vi "Swing-up Control.vi"() -> ()   [LabVIEW 2019]
uses:
  <vilib>/Simulation/Scripting/Companion Diagram/SimConfigNode/SimParams.ctl
  <vilib>/Simulation/Scripting/Companion Diagram/SimConfigNode/_simSolvers.ctl
  <vilib>/Simulation/Implementation/Shared/SIMSCR Execution Mode.ctl
  <vilib>/Platform/TimedLoop/XDataNode/timing_clust.ctl
  <vilib>/Platform/TimedLoop/XDataNode/nitl_modes.ctl
  <vilib>/Platform/TimedLoop/XDataNode/wakeup.ctl
  <vilib>/Simulation/Param Hierarchy/Typedefs/SIMPH Param Control Actions.ctl
  <vilib>/Simulation/Implementation/Shared/NILVSim_ParamChanged.vi
  <vilib>/Simulation/Implementation/Shared/NILVSim_FinishedLate.vi
  <vilib>/Simulation/Implementation/Shared/NILVSIM_BeginStep.vi
  <vilib>/Simulation/Utility/Implementation/SIM Halt.vi
  <vilib>/Simulation/DataSources/Implementation/NILVSim Signal Generator.llb/SIM Signal Generator (scalar).vi
  <vilib>/Simulation/SignalDisplay/Implementation/NILVSim Time Waveform.llb/SIM Time Waveform (vector).vi
  <vilib>/Simulation/SignalDisplay/Implementation/NILVSim Time Waveform.llb/SIM Time Waveform (scalar).vi
  <vilib>/Simulation/ContinuousLinear/Implementation/NILVSim Transfer Function Direct.llb/SIM Transfer Function Direct (SISO).vi
  <vilib>/Simulation/SignalArithmetic/Implementation/NILVSim Gain.llb/SIM Gain (dot product).vi
  <vilib>/Simulation/Nonlinear/Implementation/NILVSim Saturation.llb/SIM Saturation (scalar).vi
  <vilib>/Simulation/Implementation/Shared/NILVSim_Manager.vi
  <vilib>/Utility/error.llb/Clear Errors.vi
  <vilib>/Simulation/Implementation/Shared/NILVSim_FinalizeModel.vi
  <vilib>/Simulation/Implementation/Shared/SIM Unbundle Sim Info.vi
  <vilib>/Simulation/Implementation/Shared/SIMSH Read Queue.vi
  <vilib>/Simulation/Implementation/Shared/NILVSim_Initialize.vi
  SubVIs/Encoders.vi
  <vilib>/Simulation/Utility/Implementation/NILVSim Get Time and IsAcceptedStep.vi
  SubVIs/Motor.vi
  <vilib>/Simulation/Implementation/Shared/NILVSim_GetModelError.vi
  <vilib>/Simulation/Implementation/Shared/SIM Bundle Sim Info.vi
  <vilib>/Simulation/Scripting/Companion Diagram/SimConfigNode/SimDog.xnode
  SubVIs/Swing Up Energy Control.vi
  <vilib>/Platform/TimedLoop/XDataNode/XDataNode.xnode
  <vilib>/Simulation/Implementation/XNodeFramework/SimXNode/SimX.xnode
  <vilib>/Platform/TimedLoop/XDataNode/XDNodeRunTimeDep.lvlib
  <vilib>/Simulation/Implementation/Shared/NI_SIM_Implementation.lvlib
panel:
  in  "y":string="0"
  out "源端口":u16=65289
  out "源地址":u32=2887125761
  out "接收数据":string="0"
  out "错误输出 2":errorcluster caption="读取错误输出"
  out "错误输出":errorcluster caption="监听错误输出"
  in  "监听地址":string="192.168.8.144"
  in  "监听端口":u16=4096
  in  "Halt?":bool
  in  "Feedback Gain":dbl[](array[numeric])=[-3.39, 41.48, -1.38, 2.94]
  in  "Energy Control":T1={"Er (mJ)"=30.0, "mu (m/s^2/J)"=35.0, "u_max (m/s^2)"=6.0} {"u_max (m/s^2)" min=0.0 max=10.0 step=0.5; "mu (m/s^2/J)" min=0.0 max=150.0 step=5.0; "Er (mJ)" min=0.0 max=50.0 step=5.0}
  out "Pendulum Energy":waveform(dbl)(graph)={"t0"=timestamp(5.94 s since 1904-01-01), "dt"=1.0, "Y"=[29.900839839111626]}
  out "Pendulum Angle":waveform(dbl)(graph)={"t0"=timestamp(5.94 s since 1904-01-01), "dt"=1.0, "Y"=[-539.82421875]}
  in  "Signal Generator":T2={"Amplitude (deg)"=0.0, "Frequency (Hz)"=0.2} {"Frequency (Hz)" step=0.1}
  out "Pendulum Arm Angle":waveform(dbl)[](graph)=[{"t0"=timestamp(5.94 s since 1904-01-01), "dt"=1.0, "Y"=[0.0]}, {"t0"=timestamp(5.94 s since 1904-01-01), "dt"=1.0, "Y"=[4.74609375]}]
  out "Error":errorcluster={"status"=FALSE, "code"=-363017, "source"="ELVIS III v1.0 Write PWM.vi"}
  # "Engineering Trainer Boards"
  # "Controls Board"
  # "Swing-up Control"
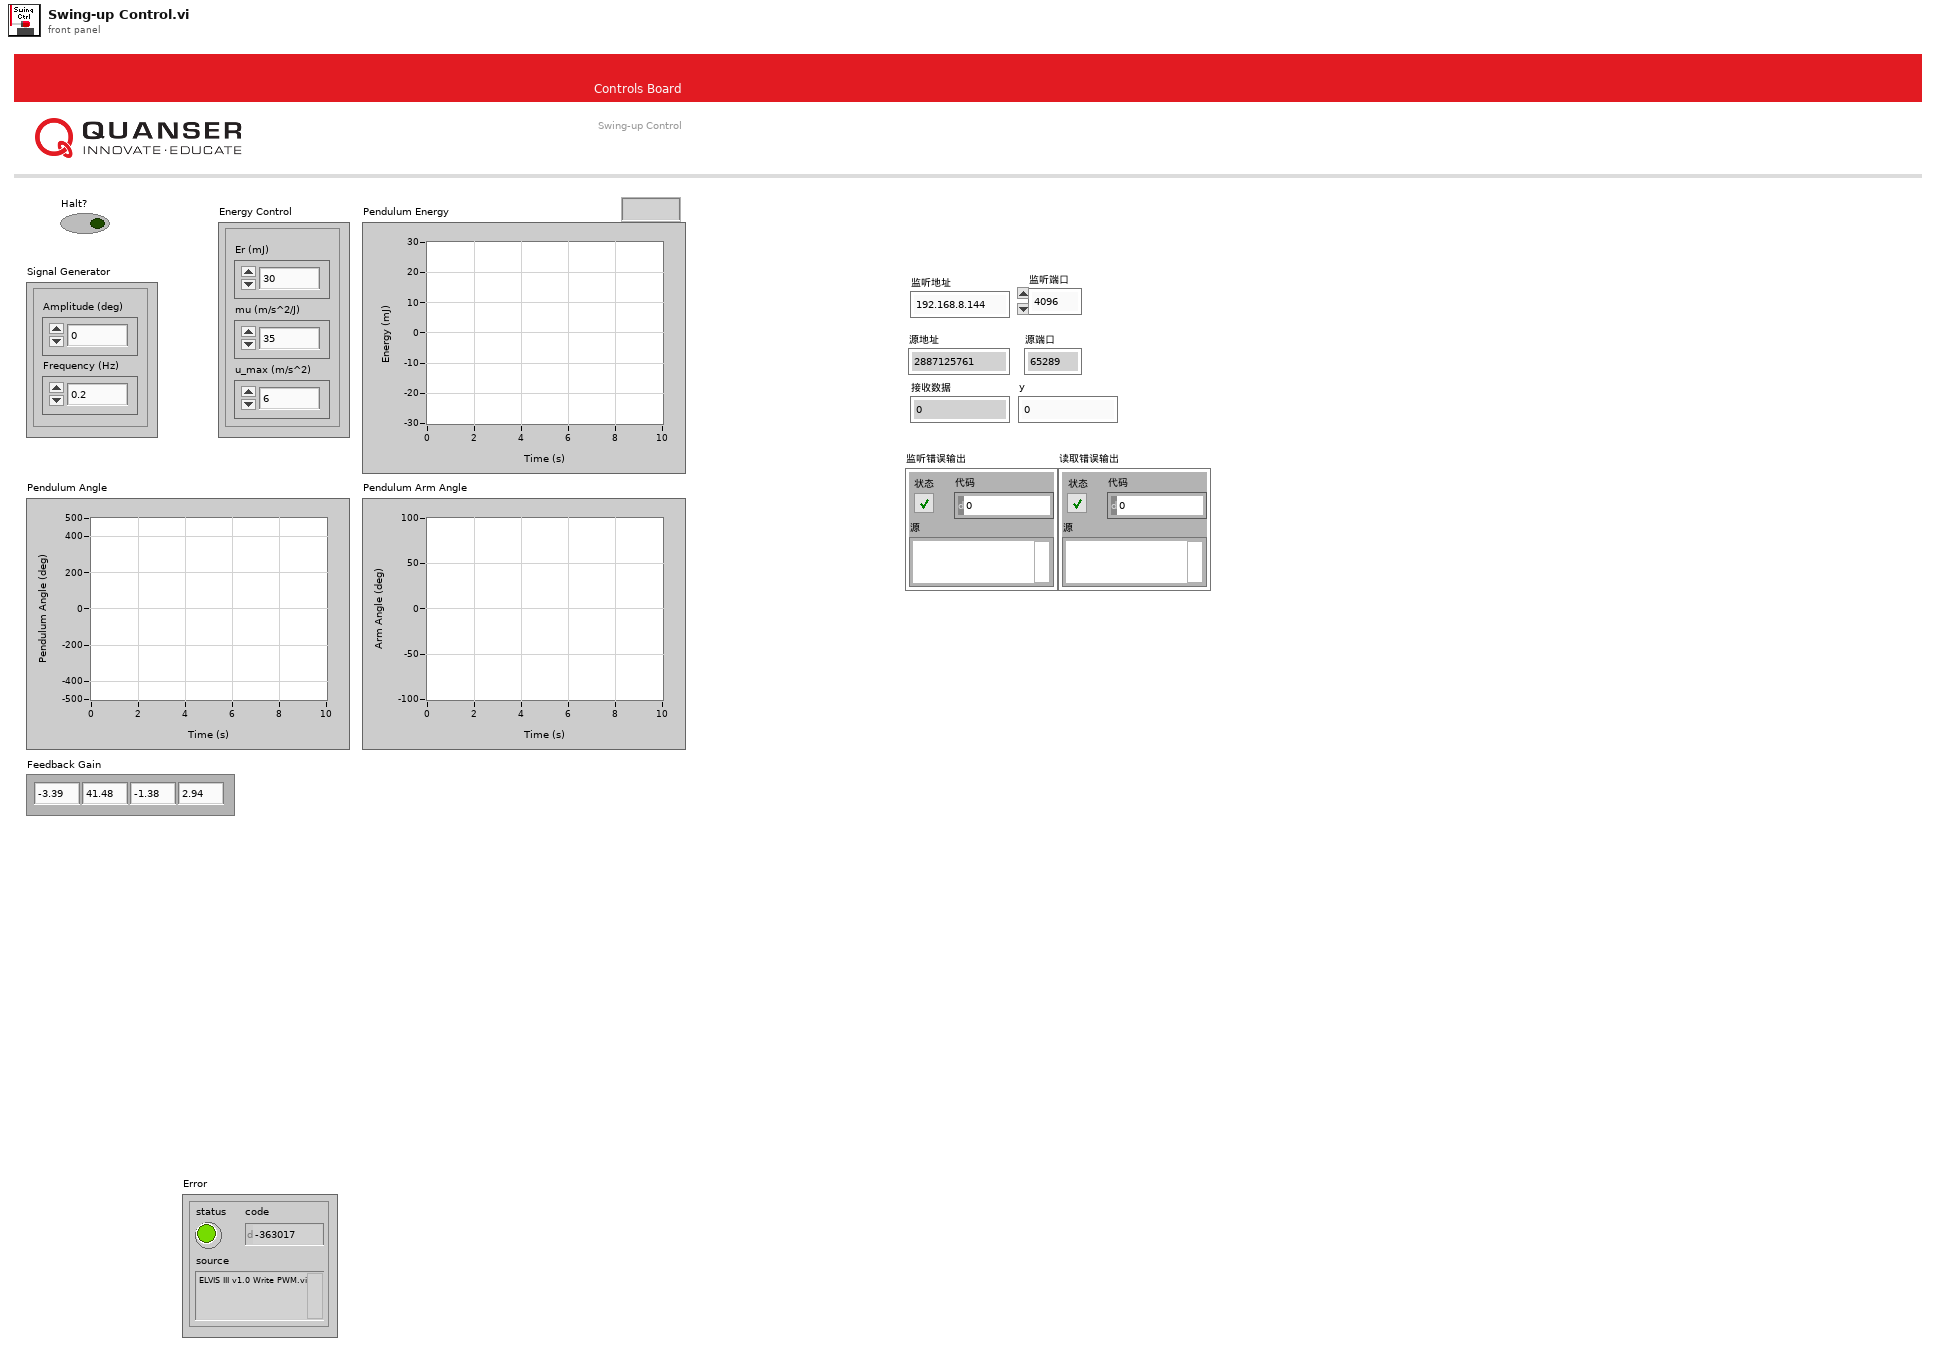
[diagram p1: front panel]
types:
  T1 = cluster{"Er (mJ)":dbl, "mu (m/s^2/J)":dbl, "u_max (m/s^2)":dbl}
  T2 = cluster{"Amplitude (deg)":dbl, "Frequency (Hz)":dbl}
  T3 = typedef "SIMSCR Execution Mode.ctl" = enum16{"Simulate to Completion", "Single Time-Step Simulation (Fixed Step Only)"}
  T4 = typedef "XDNodeRunTimeDep.lvlib/timing_clust.ctl" = cluster{"Expected End [f-1]":u64, "Actual End [f-1]":u64, "Finished Late? [f-1]":bool, "Expected End [i-1]":u64, "Actual End [i-1]":u64, "Finished Late? [i-1]":bool, "Expected Start [i]":u64, "Actual Start [i]":u64, "Expected Start [f]":u64, "Actual Start [f]":u64, "Source Name":string, "Structure Name":string, "Period":i64, "Deadline":i64, "Offset":i64, "Start":i64, "Priority":i32, "Timeout":i32, "Mode":T5, "Wakeup Reason":T6, "Error":errorcluster, "Source Type":string, "Secondary Source Type":string, "Global End Time":u64, "Global Start Time":u64, "Frame Duration":u64, "Iteration Duration":u64, "Assigned CPU":i32, "I/O Scan Engine Mode":u32}
  T5 = typedef "XDNodeRunTimeDep.lvlib/nitl_modes.ctl" = enum32{"No Change", "Process missed periods, maintain original phase", "Discard missed periods, maintain original phase", "Process missed periods, ignore original phase", "Discard missed periods, ignore original phase"}
  T6 = typedef "XDNodeRunTimeDep.lvlib/wakeup.ctl" = enum32{"Normal", "Aborted", "Asynchronous wakeup", "Timing source error", "Timed loop error", "Timeout"}
  T7 = typedef "SIMPH Param Control Actions.ctl" = enum16{"get params", "set params"}
  T8 = cluster{"SIMSH Sim Time":dbl, "x":dbl, "Multiply 2":cluster{"x*y":dbl}, "Divide 2":cluster{"x/y":dbl}, "alpha_full_dot":cluster{"output y(t)":dbl}, "Divide":cluster{"x/y":dbl}, "Negate":cluster{"-x":dbl}, "Compound Arithmetic 2":cluster{"result":dbl}, "Saturation":cluster{"output":dbl}, "Compound Arithmetic":cluster{"result":dbl}, "Subtract":cluster{"x-y":dbl}, "Multiply":cluster{"x*y":dbl}, "Sign":cluster{"-1, 0, 1":dbl}, "Cosine":cluster{"cos(x)":dbl}, "Formula Node":cluster{"E":dbl}}
  T9 = typedef "SimParams.ctl" = cluster{"Initial Time (s)":dbl, "Final Time (s)":dbl, "Step Size (s)":dbl, "ODE Solver":T10, "Minimum Step Size (s)":dbl, "Maximum Step Size (s)":dbl, "Relative Tolerance":dbl, "Absolute Tolerance":dbl, "Software Timing":bool, "Initial Step Size (s)":dbl, "Automatic Fixed Step Size?":bool, "Automatic Discrete Step Size?":bool, "Discrete Step Size (s)":dbl, "Calculate using Time Step":bool, "Solver Wired?":bool, "Prev.Frm.Expected End":u64, "Prev.Frm.Actual End":u64, "Prev.Frm.Finished Late?":bool, "Prev.Iter.Expected End":u64, "Prev.Iter.Actual End":u64, "Prev.Iter.Finished Late?":bool, "Expected Iteration Start":u64, "Actual Iteration Start":u64, "Expected Frame Start":u64, "Actual Frame Start":u64, "Source Name":string, "Name":string, "Period":i64, "Deadline":i64, "Offset":i64, "Start":i64, "Priority":i32, "Timeout":i32, "Processor":i32, "Mode":enum32{"No Change", "Process missed periods, maintain original phase", "Discard missed periods, maintain original phase", "Process missed periods, ignore original phase", "Discard missed periods, ignore original phase"}, "Wakeup reason":enum32{"Normal", "Aborted", "Asynchronous wakeup", "Timing source error", "Timed loop error", "Timeout"}, "Error":errorcluster, "Source Type":string, "Secondary Source Type":string, "Global End Time":u64, "Global Start Time":u64, "Full Solver Reset":bool, "Execution Mode":T3, "Nan/Inf Check":bool, "Custom Solver Library":string, "Solver Is Variable":bool, "custom solver name":string, "Signal Collection Decimation":u32}
  T10 = typedef "_simSolvers.ctl" = enum16{"Runge-Kutta 1 (Euler)", "Runge-Kutta 2", "Runge-Kutta 3", "Runge-Kutta 4", "Runge-Kutta 23 (variable)", "Runge-Kutta 45 (variable)", "BDF (variable)", "Adams-Moulton (variable)", "Rosenbrock (variable)", "Discrete States Only", "SDIRK 4 (variable)", "Radau 5 (variable)", "Radau 9 (variable)", "Radau 13 (variable)", "Radau [Variable Order] (variable)", "Gear's Method (variable)", "Linearizer", "State Query", "Trim Eval", "Custom Solver"}
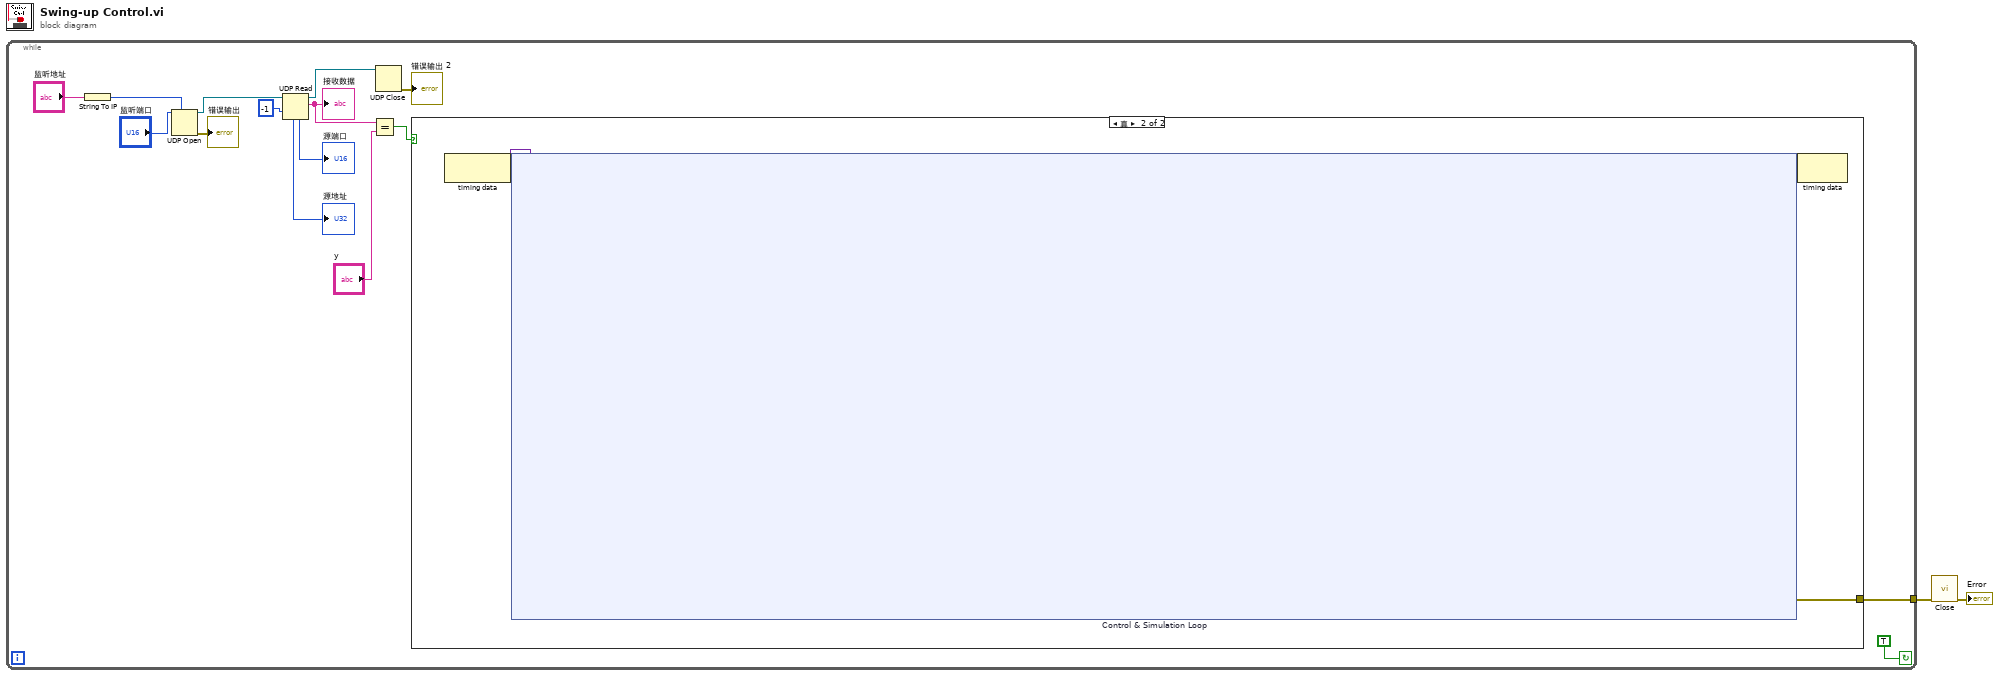
[diagram p0: block diagram]
diagram:
  n1 = while {
    tunnel: [w17] -> w1
    stop <- TRUE continue-if-true
    n2 = String To IP(1:"监听地址") -> (0:w15:u32)
    n3 = UDP Open(7:w15, 11:"监听端口") -> (port=w11:refnum<k16>, 0:→"错误输出":errorcluster)  [unwired: 3 in, 1 out]
    n4 = UDP Read(connection ID=w11, timeout ms (25000)=-1 ("超时毫秒(25000)")) -> (data out=w5:string, 3:w10:refnum<k16>, 4:→"源端口":u16, 6:→"源地址":u32)  [unwired: 2 in, 1 out]
    "接收数据" <- w5
    n5 = Equal?(x=w5, y="y") -> (x = y?=w3:bool)
    n6 = UDP Close(connection ID=w10) -> (error out=→"错误输出 2":errorcluster)  [unwired: 1 in, 1 out]
    n7 = case shown="真" w3 {
      tunnel: [_ w18] -> w17
      frame False {
      }
      frame True {
        n8 = node-c288() -> (w20:variant)  [unwired: 1 in]
        n9 = node-c254 "Control & Simulation Loop"(w20) -> (w19:variant, w18:errorcluster)
        n10 = node-c288(w19) -> ()  [unwired: 1 out]
      }
    }
  }
  n11 = call "Close.vi"("error in"=w1) -> ("error out"=→"Error":errorcluster)  [unwired: 10 in]
